vi "Smite All.vi"(8 "Error In":errorcluster) -> (0 "Error Out":errorcluster)   [LabVIEW 2018, in "Bookmark Manager.lvlib" / "Tests.lvlib"]
uses:
  Tests.lvlib
  <vilib>/addons/_JKI Toolkits/Caraya/classes/Test/Test.lvclass
  Bookmark Manager.lvlib
  Toolkit/Toolkit.lvlib
  <vilib>/addons/_JKI Toolkits/Caraya/classes/Assert/Assert.lvclass
  tests/Tests.lvlib
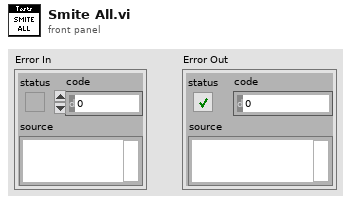
[diagram p1: front panel]
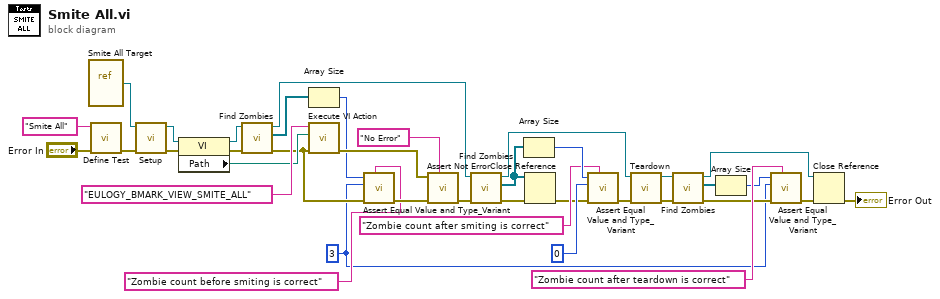
[diagram p0: block diagram]
diagram:
  w1 = 3 ("size(s)")
  n1 = vi-ref "Smite All Target.vi"() -> (w34:refnum<vi>)
  n2 = call <vilib>:"Define Test.vi"("error in (no error)"="Error In", "Label (VI Title)"="Smite All") -> ("error out"=w35:errorcluster)  [unwired: 9 in]
  n3 = call "Setup.vi"("Error In"=w35, "VI In"=w34) -> ("Error Out"=w32:errorcluster, "VI Out"=w31:refnum<vi>)  [unwired: 8 in]
  n4 = property class="VI"(reference=w31, error in=w32) -> (reference out=w8:refnum<vi>, error out=w9:errorcluster, "Path"=w18:path)
  n5 = call "Find Zombies.vi"("Error In"=w9, "VI In"=w8) -> ("Error Out"=w5:errorcluster, "Graves"=w6:refnum<vi>[], "VI Out"=w7:refnum<vi>)  [unwired: 7 in]
  n6 = Array Size(array=w6) -> (size(s)=w2:i32)
  n7 = call "Execute VI Action.vi"("Error In"=w5, "VI"=w18, "Menu Tag"="EULOGY_BMARK_VIEW_SMITE_ALL") -> ("Error Out"=w26:errorcluster)  [unwired: 8 in]
  n8 = call <vilib>:"Assert Equal Value and Type_Variant.vi"("Label"="Zombie count before smiting is correct", "error in (no error)"=w5, "Y"=w1, "X"=w2) -> ("error out"=w4:errorcluster)  [unwired: 7 in]
  n9 = call <vilib>:"Assert Not Error.vi"("Label"="No Error", "error in (no error)"=w4, "Not Error?"=w26) -> ("error out"=w25:errorcluster)  [unwired: 8 in]
  n10 = call "Find Zombies.vi"("Error In"=w25, "VI In"=w7) -> ("Error Out"=w28:errorcluster, "Graves"=w19:refnum<vi>[], "VI Out"=w23:refnum<vi>)  [unwired: 7 in]
  n11 = Array Size(array=w19) -> (size(s)=w30:i32)
  n12 = Close Reference(reference=w19, error in (no error)=w28) -> (error out=w20:errorcluster)
  n13 = call <vilib>:"Assert Equal Value and Type_Variant.vi"("Label"="Zombie count after smiting is correct", "error in (no error)"=w20, "Y"=0 ("size(s)"), "X"=w30) -> ("error out"=w24:errorcluster)  [unwired: 7 in]
  n14 = call "Teardown.vi"("Error In"=w24, "VI In"=w23) -> ("Error Out"=w16:errorcluster, "VI Out"=w15:refnum<vi>)  [unwired: 8 in]
  n15 = call "Find Zombies.vi"("Error In"=w16, "VI In"=w15) -> ("Error Out"=w13:errorcluster, "Graves"=w11:refnum<vi>[], "VI Out"=w14:refnum<vi>)  [unwired: 7 in]
  n16 = Array Size(array=w11) -> (size(s)=w10:i32)
  n17 = call <vilib>:"Assert Equal Value and Type_Variant.vi"("Label"="Zombie count after teardown is correct", "error in (no error)"=w13, "Y"=w1, "X"=w10) -> ("error out"=w12:errorcluster)  [unwired: 7 in]
  n18 = Close Reference(reference=w14, error in (no error)=w12) -> (error out=→"Error Out":errorcluster)
